vi "Get Value.vi"(8 "error in (no error)":errorcluster, 11 "Cell Context in":refnum<class "Cell Context.lvclass">) -> (0 "error out":errorcluster, 2 "Value":variant, 3 "Cell Context out":refnum<class "Cell Context.lvclass">)   [LabVIEW 2024, in "SourceGrid.lvlib" / "Cell Context.lvclass"]
uses:
  Cell Context.lvclass
  Cell Context.lvclass/Cell Context.ctl
  D:/git/Sourcegrid-LabVIEW/dll/SourceGrid.dll
  dll/SourceGrid.dll
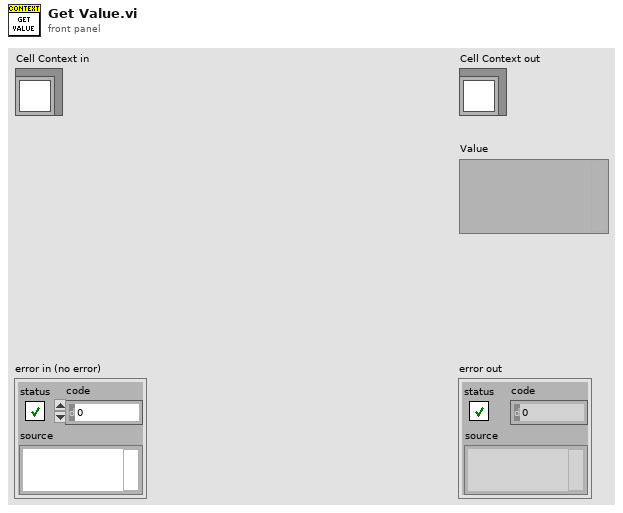
[diagram p1: front panel]
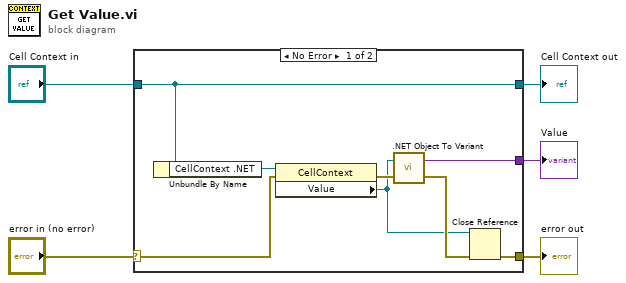
[diagram p0: block diagram]
diagram:
  n1 = case shown="No Error" "error in (no error)" {
    selector: "error in (no error)" -> [w11 w14]
    tunnel: [w7 w14] -> w4
    tunnel: [w13 w15] -> w2
    tunnel: "Cell Context in" -> [w13 w15]
    tunnel: [w8 _] -> w1
    frame No Error {
      n2 = Unbundle By Name(w13) -> ("CellContext .NET"=w12:refnum<k24>)
      n3 = property class="CellContext"(reference=w12, error in=w11) -> (error out=w10:errorcluster, "Value"=w6:refnum<k24>)  [unwired: 1 out]
      n4 = call <vilib>:".NET Object To Variant.vi"("error in (no error)"=w10, ".NET object"=w6) -> ("error out"=w9:errorcluster, "variant"=w8:variant)
      n5 = Close Reference(reference=w6, error in (no error)=w9) -> (error out=w7:errorcluster)
    }
    frame Error {
    }
  }
  "error out" <- w4
  "Cell Context out" <- w2
  "Value" <- w1
